vi "Modbus Life Bit Toggle.vi"(0 "FVIR Boolean Array Input":bool[](array[boolean]), 1 "Modbus master in":refnum<class "Modbus Master.lvclass">, 2 "UI":refnum<queue>, 5 "seconds since 1Jan1904 in":timestamp, 9 "Toggle Input":bool, 11 "error in (no error)":errorcluster) -> (3 "Modbus master out":refnum<class "Modbus Master.lvclass">, 4 "FV Output":bool[](array[boolean]), 6 "seconds since 1Jan1904 out":timestamp, 10 "Toggle Output":bool, 14 "FV Output Value":u32, 15 "error out":errorcluster)   [LabVIEW 2023, in "Modbus.lvlib"]
uses:
  Modbus.lvlib
  <vilib>/NI/Modbus Library/API/Master/Modbus Master.lvclass
  support/Message Queue/Message Cluster.ctl
  support/Message Queue/Enqueue Message (Single).vi
  support/Message Queue/Message Queue.lvlib
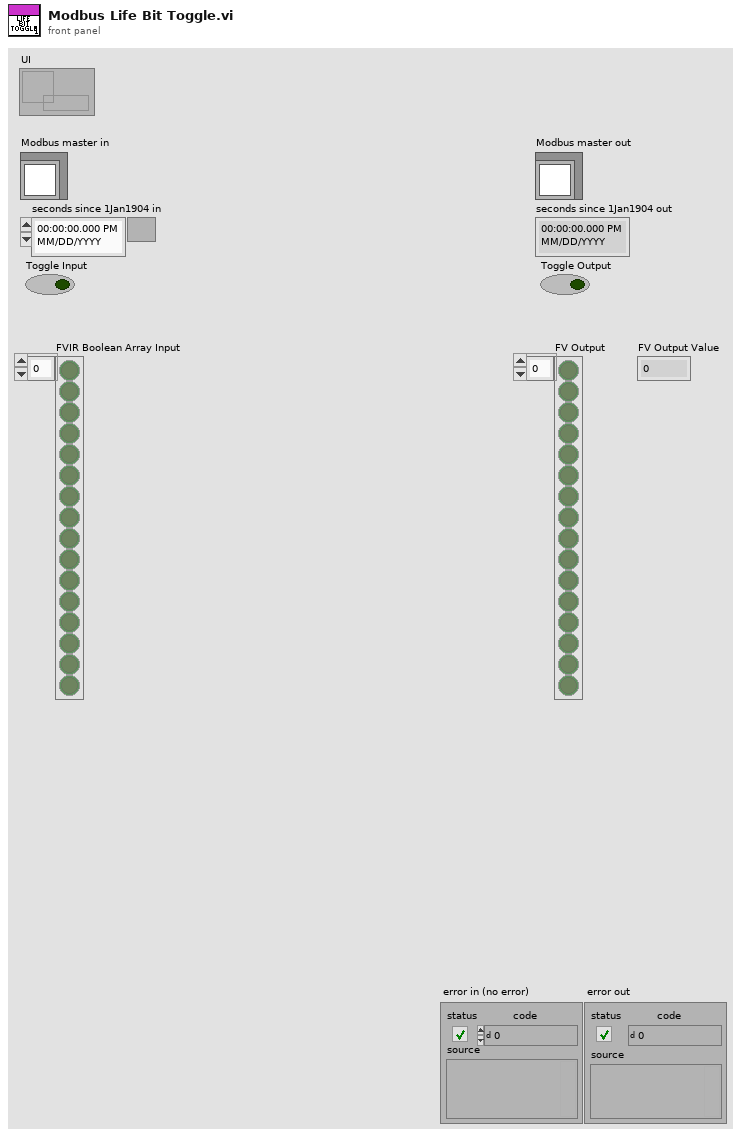
[diagram p1: front panel]
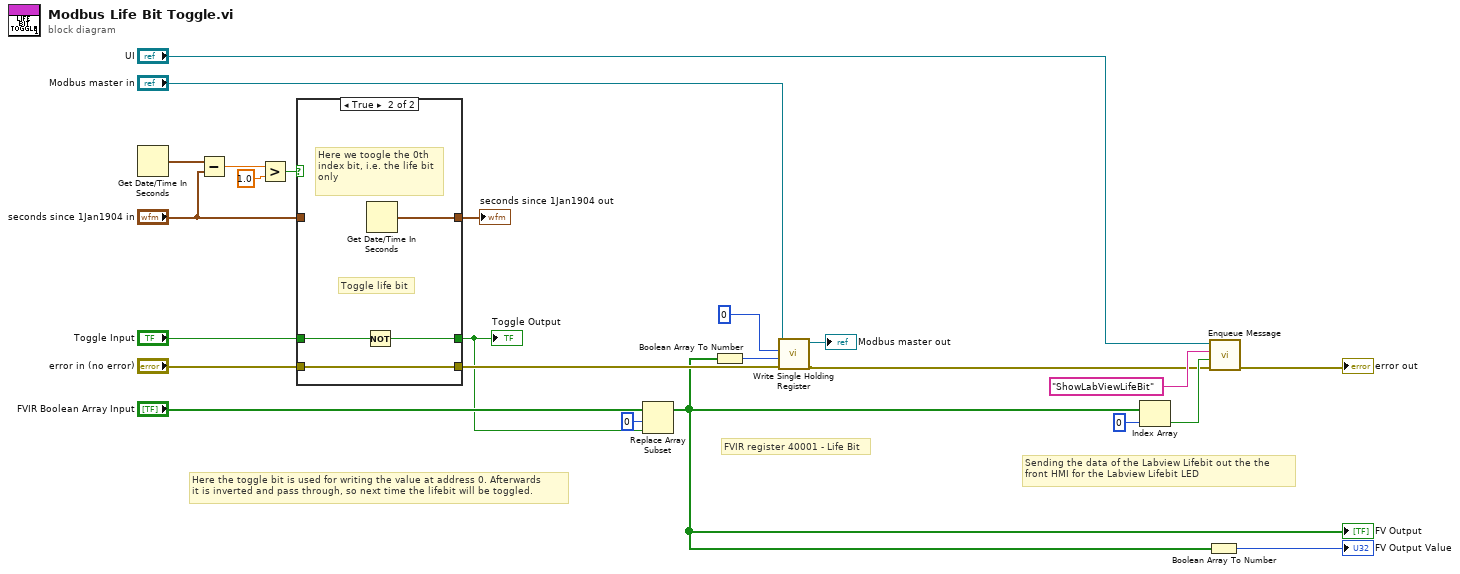
[diagram p0: block diagram]
diagram:
  # "Sending the data of the Labview Lifebit out the the \nfront HMI for the Labview Lifebit LED"
  # "Here the toggle bit is used for writing the value at address 0. Afterwards\nit is inverted and pass through, so next time the lifebit will be toggled."
  # "FVIR register 40001 - Life Bit"
  n1 = Get Date/Time In Seconds() -> (seconds since 1Jan1904=w18:timestamp)
  n2 = Subtract(x=w18, y="seconds since 1Jan1904 in") -> (x-y=w19:dbl)
  n3 = Greater?(x=w19, y=1.0) -> (0:w21:bool)
  n4 = case shown="True" w21 {
    tunnel: "seconds since 1Jan1904 in" -> [w26 _]
    tunnel: [w26 w31] -> w22
    tunnel: "Toggle Input" -> [w27 w30]
    tunnel: [w27 w29] -> w8
    tunnel: "error in (no error)" -> [w25 w28]
    tunnel: [w25 w28] -> w9
    frame False {
    }
    frame True {
      # "Toggle life bit"
      # "Here we toogle the 0th index bit, i.e. the life bit only"
      n5 = Not(x=w30) -> (.not. x?=w29:bool)
      n6 = Get Date/Time In Seconds() -> (seconds since 1Jan1904=w31:timestamp)
    }
  }
  "Toggle Output" <- w8
  "seconds since 1Jan1904 out" <- w22
  n7 = Replace Array Subset(array="FVIR Boolean Array Input", new element=w8, index=0) -> (w1:bool[])
  "FV Output" <- w1
  n8 = Boolean Array To Number(Boolean array=w1) -> (number=w17:u32)
  n9 = call-dynamic "Write Single Holding Register.vi"("error in"=w9, "register to write"=w17, "address"=u16 0 ("starting address"), "Modbus master in"="Modbus master in") -> ("error out"=w3:errorcluster, "Modbus master out"=→"Modbus master out":refnum<class "Modbus Master.lvclass">)  [unwired: 6 in]
  n10 = Index Array(array=w1, index=0) -> (element=w7:bool)
  n11 = Boolean Array To Number(Boolean array=w1) -> (number=→"FV Output Value":u32)
  n12 = call-poly "Enqueue Message.vi"("error in (no error)"=w3, "Message Data"=w7, "Message"="ShowLabViewLifeBit", "Message Queue"="UI") -> ("error out"=→"error out":errorcluster)  [unwired: 6 in, 1 out]
